vi "AddTreeItem1.vi"(5 "CtlRef 2":refnum<vi>, 6 "error in":errorcluster, 7 "folder names":string[](array[string]), 8 "filenames":string[](array[string]), 9 "path":path) -> (0 "error out":errorcluster, 1 "PathArray":path[](array[path]), 3 "path out":path, 4 "CtlRef 3":refnum<vi>)   [LabVIEW 2010]
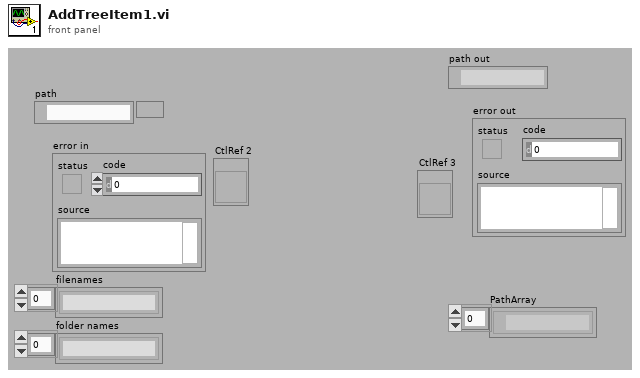
[diagram p1: front panel]
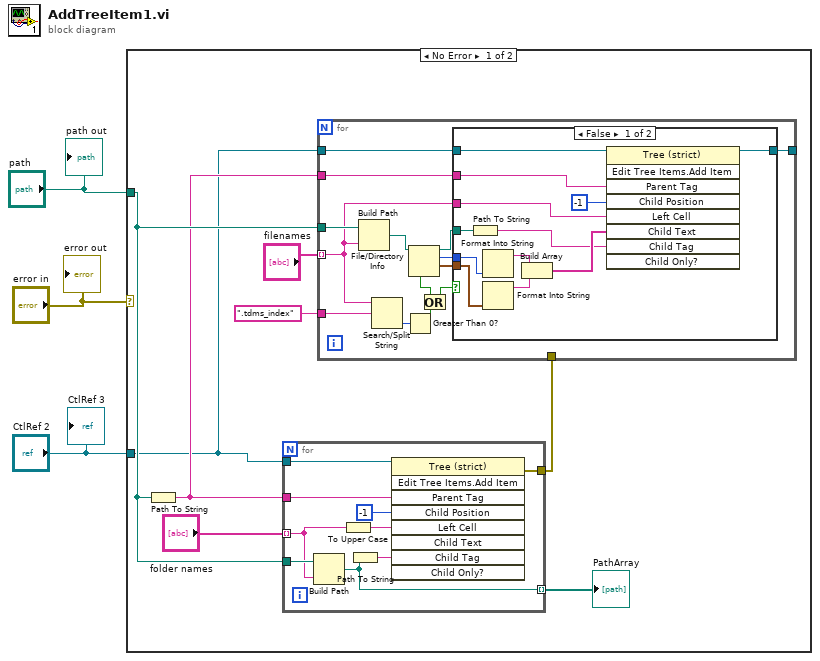
[diagram p0: block diagram]
diagram:
  n1 = case shown="No Error" "error in" {
    tunnel: "path" -> [w7 _]
    tunnel: "CtlRef 2" -> [w4 _]
    frame No Error {
      n2 = Path To String(path=w7) -> (string=w6:string)
      n3 = for {
        tunnel: "folder names" -> [w46] mode=indexing
        tunnel: w7 -> [w47]
        tunnel: [w45] -> w11 mode=indexing
        tunnel: w6 -> [w44]
        tunnel: w4 -> [w40]
        tunnel: [w39] -> w5
        n4 = Build Path(base path=w47, name or relative path=w46) -> (appended path=w45:path)
        n5 = To Upper Case(1:w46) -> (0:w42:string)
        n6 = Path To String(path=w45) -> (string=w41:string)
        n7 = invoke class="Tree (strict)" method="Edit Tree Items.Add Item"(reference=w40, "Parent Tag"=w44, "Child Position"=-1, "Left Cell"=w42, "Child Tag"=w41) -> (error out=w39:errorcluster)  [unwired: 4 in, 8 out]
      }
      "PathArray" <- w11
      n8 = for {
        tunnel: "filenames" -> [w20] mode=indexing
        tunnel: w7 -> [w25]
        tunnel: ".tdms_index" -> [w19]
        tunnel: w6 -> [w14]
        tunnel: w4 -> [w13]
        tunnel: [w12] -> _
        tunnel: w5 -> [_]
        n9 = Build Path(base path=w25, name or relative path=w20) -> (appended path=w21:path)
        n10 = Search/Split String(string=w20, search string/char (-)=w19) -> (offset of match=w18:i32)  [unwired: 1 in, 2 out]
        n11 = Greater Than 0?(x=w18) -> (x > 0?=w17:bool)
        n12 = File/Directory Info(path=w21) -> (path out=w22:path, size=w23:i64, last mod=w24:timestamp, shortcut=w16:bool)  [unwired: 1 in, 3 out]
        n13 = Or(x=w16, y=w17) -> (x .or. y?=w15:bool)
        n14 = case shown="False" w15 {
          tunnel: w24 -> [w36 _]
          tunnel: w23 -> [w37 _]
          tunnel: w20 -> [w30 _]
          tunnel: w22 -> [w33 _]
          tunnel: w14 -> [w32 _]
          tunnel: w13 -> [w27 w38]
          tunnel: [w26 w38] -> w12
          frame False {
            n15 = Path To String(path=w33) -> (string=w28:string)
            n16 = Format Into String(w37) -> (resulting string=w34:string)  [unwired: 3 in, 1 out]
            n17 = Format Into String(w36) -> (resulting string=w35:string)  [unwired: 3 in, 1 out]
            n18 = Build Array(w34, w35) -> (w29:string[])
            n19 = invoke class="Tree (strict)" method="Edit Tree Items.Add Item"(reference=w27, "Parent Tag"=w32, "Child Position"=-1 ("dimension size"), "Left Cell"=w30, "Child Text"=w29, "Child Tag"=w28) -> (reference out=w26:refnum<vi>)  [unwired: 3 in, 8 out]
          }
          frame True {
          }
        }
      }
    }
    frame Error {
    }
  }
  "error out" <- "error in"
  "path out" <- "path"
  "CtlRef 3" <- "CtlRef 2"
